vi "DSF.Engine.Execution.Framework.Initialize.vi"(8 "error in (no error)":errorcluster, 10 "Framework Configuration":refnum<class "DSF.Shared.Configuration.Framework.lvclass">, 11 "Framework in":refnum<class "DSF.Engine.Execution.Framework.lvclass">) -> (0 "error out":errorcluster, 3 "Framework out":refnum<class "DSF.Engine.Execution.Framework.lvclass">)   [LabVIEW 2016, in "DSF.Engine.lvlib" / "DSF.Engine.Execution.Framework.lvclass"]
uses:
  DSF.Engine.Execution.Framework.lvclass
  Shared/Classes/Framework/DSF.Shared.Configuration.Framework.lvclass
  <vilib>/NI Veristand/Custom Device API/Custom Device Item Ref.ctl
  <vilib>/NI Veristand/Custom Device API/Custom Device API.lvlib
panel:
  in  "Device Item Ref":T1=18446744073709551615 format="%.0x"
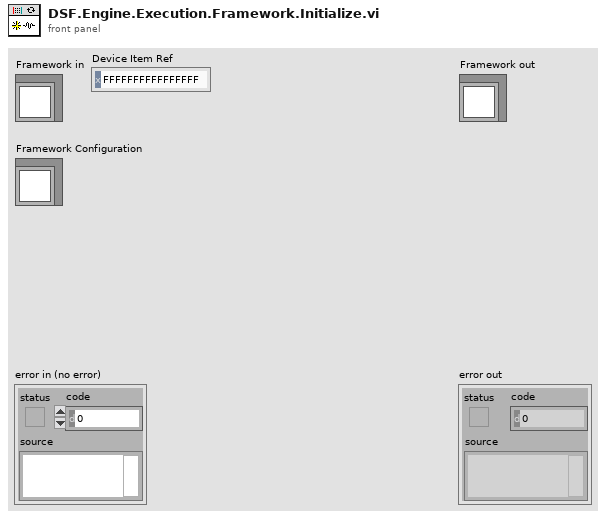
[diagram p1: front panel]
types:
  T1 = typedef "Custom Device API.lvlib/Custom Device Item Ref.ctl" = u64
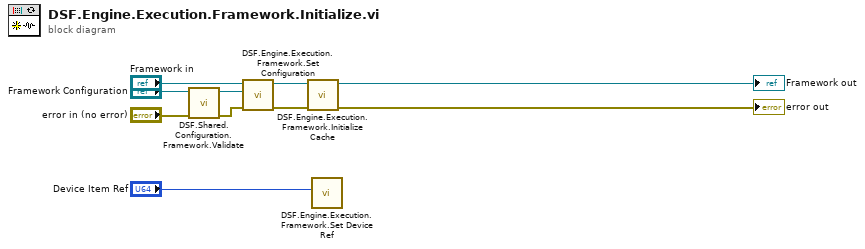
[diagram p0: block diagram]
diagram:
  n1 = call "DSF.Shared.Configuration.Framework.Validate.vi"("error in (no error)"="error in (no error)", "Framework Configuration in"="Framework Configuration") -> ("error out"=w7:errorcluster, "Framework Configuration out"=w6:refnum<class "DSF.Shared.Configuration.Framework.lvclass">)  [unwired: 8 in]
  n2 = call "DSF.Engine.Execution.Framework.Set Configuration.vi"("error in (no error)"=w7, "Framework Configuration"=w6, "Framework in"="Framework in") -> ("error out"=w4:errorcluster, "Framework out"=w5:refnum<class "DSF.Engine.Execution.Framework.lvclass">)  [unwired: 7 in]
  n3 = call "DSF.Engine.Execution.Framework.Initialize Cache.vi"("error in (no error)"=w4, "Framework in"=w5) -> ("error out"=→"error out":errorcluster, "Framework out"=→"Framework out":refnum<class "DSF.Engine.Execution.Framework.lvclass">)  [unwired: 8 in]
  n4 = call "DSF.Engine.Execution.Framework.Set Device Ref.vi"("Device Item Ref"="Device Item Ref") -> ()  [unwired: 9 in, 2 out]
